vi "SUB-Interval_Realtime-Average.vi"(7 "Mode":enum16{"Add", "Reset"}(ring), 11 "Input":dbl format="%#.2g") -> (3 "Average":dbl format="%#.2g")   [LabVIEW 2015]
panel:
  out "Count":u32=1
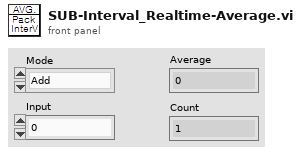
[diagram p1: front panel]
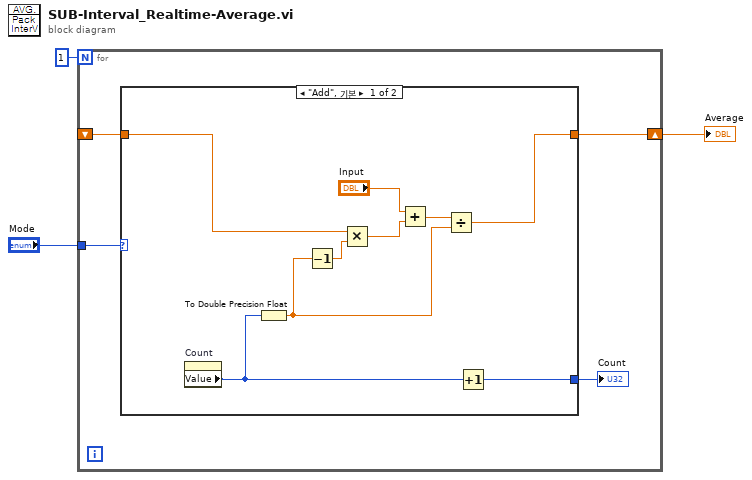
[diagram p0: block diagram]
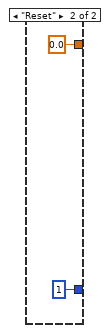
[diagram p2: hidden frame]
diagram:
  n1 = for {
    N: 1 -> [_]
    tunnel: "Mode" -> [w7]
    shift-right: [w6] -> w1
    shift-left: _ -> [w5]
    n2 = case shown="\"Add\", 기본" w7 {
      tunnel: [w11 0.0] -> w6
      tunnel: w5 -> [w10 _]
      tunnel: [w9 u32 1] -> w4
      frame "Add", Default {
        n3 = property on="Count" class="DigNum (엄격한)"() -> ("Value"=w8:u32)  [unwired: 2 in, 2 out]
        n4 = To Double Precision Float(number=w8) -> (double precision float=w12:dbl)
        n5 = Decrement(x=w12) -> (x-1=w15:dbl)
        n6 = Multiply(x=w10, y=w15) -> (x*y=w13:dbl)
        n7 = Add(x="Input", y=w13) -> (x+y=w14:dbl)
        n8 = Divide(x=w14, y=w12) -> (x/y=w11:dbl)
        n9 = Increment(x=w8) -> (x+1=w9:u32)
      }
      frame "Reset" {
      }
    }
    "Count" <- w4
  }
  "Average" <- w1
